vi "Read Scale.vi"(8 "error in (no error)":errorcluster, 11 "Slide.lvclass in":refnum<class "Slide.lvclass">) -> (0 "error out":errorcluster, 2 "Scale":refnum<vi>, 3 "Slide.lvclass out":refnum<class "Slide.lvclass">)   [LabVIEW 2015, in "Slide.lvclass"]
uses:
  Slide.lvclass
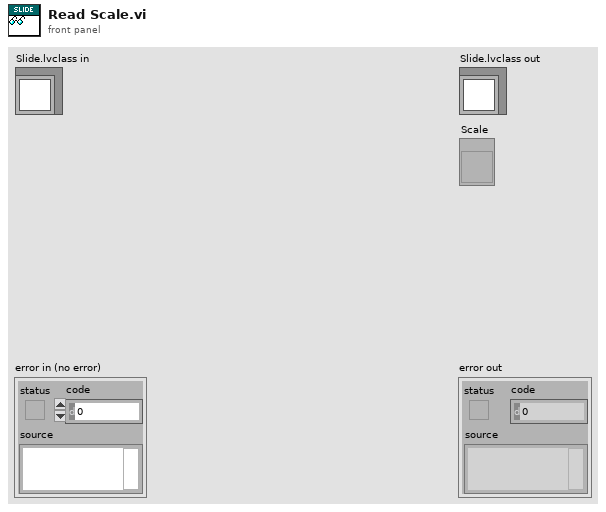
[diagram p1: front panel]
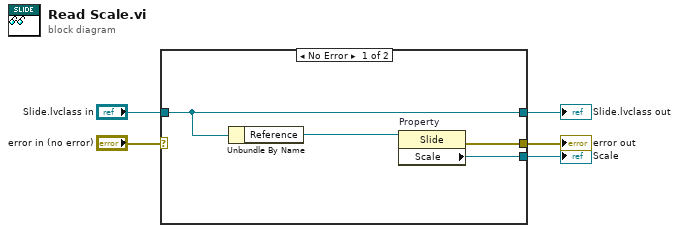
[diagram p0: block diagram]
diagram:
  n1 = case shown="No Error" "error in (no error)" {
    selector: "error in (no error)" -> [_ w11]
    tunnel: [w8 w11] -> w4
    tunnel: [w7 w10] -> w2
    tunnel: "Slide.lvclass in" -> [w7 w10]
    tunnel: [w9 _] -> w1
    frame No Error {
      n2 = Unbundle By Name(w7) -> ("Reference"=w6:refnum<vi>)
      n3 = property on="Property" class="Slide"(reference=w6) -> (error out=w8:errorcluster, "Scale"=w9:refnum<vi>)  [unwired: 1 in, 1 out]
    }
    frame Error {
    }
  }
  "error out" <- w4
  "Slide.lvclass out" <- w2
  "Scale" <- w1
